vi "Read Vsp.vi"(8 "error in":errorcluster, 11 "Session HVPS in":refnum<class "Session HVPS.lvclass">) -> (0 "error out":errorcluster, 2 "Vsp":dbl, 3 "Session HVPS out":refnum<class "Session HVPS.lvclass">)   [LabVIEW 2014, in "Session HVPS.lvclass"]
uses:
  Session HVPS.lvclass
  Session HVPS.lvclass/Session HVPS.ctl
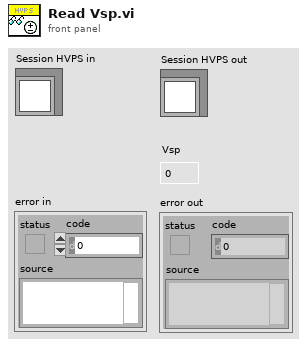
[diagram p1: front panel]
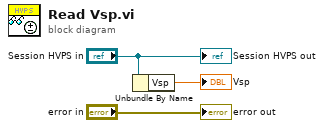
[diagram p0: block diagram]
diagram:
  n1 = Unbundle By Name("Session HVPS in") -> ("Vsp"=→"Vsp":dbl)
  "error out" <- "error in"
  "Session HVPS out" <- "Session HVPS in"
